vi "RegisterEvents.vi"(8 "Error In":errorcluster, 10 "Root Actor's Enqueuer":refnum<class "Message Enqueuer.lvclass">, 11 "Nested Actor's EnqueuerArray":refnum<class "Message Enqueuer.lvclass">[](array[class])) -> (0 "Error Out":errorcluster)   [LabVIEW 2019, in "TestBench.lvlib" / "TestBench.lvclass"]
uses:
  TestBench.lvclass
  <vilib>/ActorFramework/Message Enqueuer/Message Enqueuer.lvclass
  UserManagement/UserManagement/UserInfo.lvclass
  C:/Program Files (x86)/National Instruments/LabVIEW 2019/vi.lib/NI/Event Source Actor/Event Source/Event/Event.lvclass
  TestBench Messages/SetPrivileges Msg/SetPrivileges Msg.lvclass
  C:/Program Files (x86)/National Instruments/LabVIEW 2019/vi.lib/NI/Event Source Actor/Event Source/Event Source Messages/Event Generated Msg/Event Generated Msg.lvclass
  TestSetup/TestSetup/TestConfiguration.lvclass
  TestBench Messages/Write TestConfiguration Msg/Write TestConfiguration Msg.lvclass
  SoftwareSetup/SoftwareSetup/StationOptions.lvclass
  TestBench Messages/Write StationOptions Msg/Write StationOptions Msg.lvclass
  HardwareSetup_model001/HardwareSetup_modle001/InstrumentCommunication.lvclass
  TestBench Messages/Write InstrumentCommunication Msg/Write InstrumentCommunication Msg.lvclass
  SystemSetup/SystemSetup/SystemConfiguration.lvclass
  TestBench Messages/SystemConfigChanged Msg/SystemConfigChanged Msg.lvclass
  LocalReport/LocalReport/TestReport.lvclass
  TestBench Messages/Write ShortTestReport Msg/Write ShortTestReport Msg.lvclass
  SignalProcessing/SignalProcessing/LunchTest.lvclass
  TestBench Messages/Write Fixture ID Msg/Write Fixture ID Msg.lvclass
  DataBase/DataBase/MySQL initial error.lvclass
  TestBench Messages/Reconnection MySQL Msg/Reconnection MySQL Msg.lvclass
  SignalProcessing/SignalProcessing/Exit.lvclass
  TestBench Messages/Exit Msg/Exit Msg.lvclass
  <vilib>/NI/Event Source Actor/Event Source/Event/Event.lvclass/Event.ctl
  <vilib>/NI/Event Source Actor/Event Source/Event Source Messages/Register Msg/Register Msg.lvclass/Register Msg.ctl
  <vilib>/ActorFramework/Message Enqueuer/Message Enqueuer.lvclass/Message Enqueuer.ctl
  <vilib>/ActorFramework/Message Enqueuer/Enqueue.vi
  <vilib>/NI/Event Source Actor/Event Source/Event Source Messages/Register Msg/Register Msg.lvclass
  C:/Program Files (x86)/National Instruments/LabVIEW 2019/vi.lib/ActorFramework/Message/Message.lvclass
  <vilib>/ActorFramework/Message Priority Queue/Priority Enqueue.vi
  <vilib>/NI/Event Source Actor/Event Source/Event/Event.lvclass
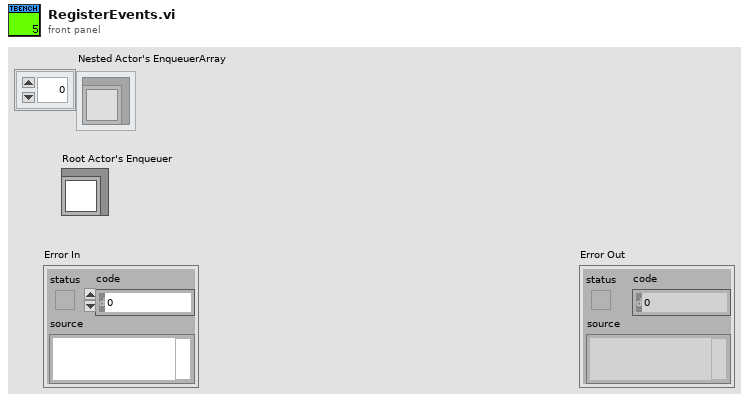
[diagram p1: front panel]
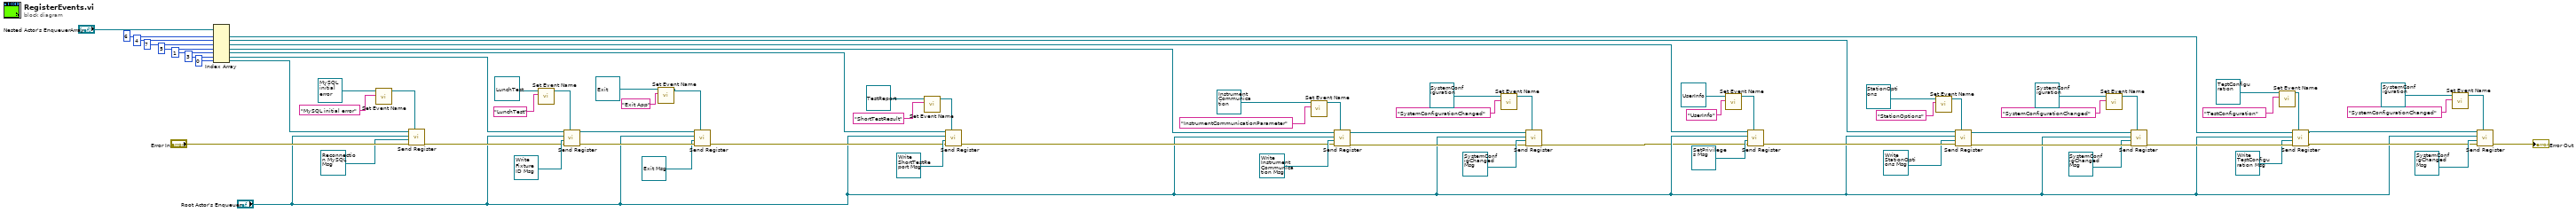
[diagram p0: block diagram]
diagram:
  n1 = Index Array(array="Nested Actor's EnqueuerArray", index #1=6 ("index"), index #2=4 ("index"), index #3=7 ("index"), index #4=5 ("index"), index #5=1 ("index"), index #6=3 ("index"), index #7=0 ("index")) -> (element #1=w67:refnum<class "Message Enqueuer.lvclass">, element #2=w68:refnum<class "Message Enqueuer.lvclass">, element #3=w69:refnum<class "Message Enqueuer.lvclass">, element #4=w4:refnum<class "Message Enqueuer.lvclass">, element #5=w3:refnum<class "Message Enqueuer.lvclass">, element #6=w2:refnum<class "Message Enqueuer.lvclass">, element #7=w1:refnum<class "Message Enqueuer.lvclass">)
  n2 = call <vilib>:"Set Event Name.vi"("Name (Generic)"="MySQL initial error", "Event In"=refnum<class "MySQL initial error.lvclass"> refnum ("DataBase.lvlib:MySQL initial erroe.lvclass")) -> ("Event Out"=w21:refnum<class "MySQL initial error.lvclass">)  [unwired: 9 in]
  n3 = call <vilib>:"Send Register.vi"("Event"=w21, "Error In"="Error In", "Event Handler"=refnum<class "Reconnection MySQL Msg.lvclass"> refnum ("TestBench.lvlib:Reconnection MySQL Msg.lvclass"), "Registrant Address"="Root Actor's Enqueuer", "Event Source Address"=w1) -> ("Error Out"=w19:errorcluster)  [unwired: 5 in, 1 out]
  n4 = call <vilib>:"Set Event Name.vi"("Name (Generic)"="LunchTest", "Event In"=refnum<class "LunchTest.lvclass"> refnum ("SignalProcessing.lvlib:LunchTest.lvclass")) -> ("Event Out"=w25:refnum<class "LunchTest.lvclass">)  [unwired: 9 in]
  n5 = call <vilib>:"Send Register.vi"("Event"=w25, "Error In"=w19, "Event Handler"=refnum<class "Write Fixture ID Msg.lvclass"> refnum ("TestBench.lvlib:Write Fixture ID Msg.lvclass"), "Registrant Address"="Root Actor's Enqueuer", "Event Source Address"=w2) -> ("Error Out"=w16:errorcluster, "Event Source Address Out"=w15:refnum<class "Message Enqueuer.lvclass">)  [unwired: 5 in]
  n6 = call <vilib>:"Set Event Name.vi"("Name (Generic)"="Exit App", "Event In"=refnum<class "Exit.lvclass"> refnum ("SignalProcessing.lvlib:Exit.lvclass")) -> ("Event Out"=w12:refnum<class "Exit.lvclass">)  [unwired: 9 in]
  n7 = call <vilib>:"Send Register.vi"("Event"=w12, "Event Handler"=refnum<class "Exit Msg.lvclass"> refnum ("TestBench.lvlib:Exit Msg.lvclass"), "Registrant Address"="Root Actor's Enqueuer", "Event Source Address"=w15) -> ()  [unwired: 6 in, 2 out]
  n8 = call <vilib>:"Set Event Name.vi"("Name (Generic)"="ShortTestResult", "Event In"=refnum<class "TestReport.lvclass"> refnum ("LocalReport.lvlib:TestReport.lvclass")) -> ("Event Out"=w29:refnum<class "TestReport.lvclass">)  [unwired: 9 in]
  n9 = call <vilib>:"Send Register.vi"("Event"=w29, "Error In"=w16, "Event Handler"=refnum<class "Write ShortTestReport Msg.lvclass"> refnum ("TestBench.lvlib:Write ShortTestReport Msg.lvclass"), "Registrant Address"="Root Actor's Enqueuer", "Event Source Address"=w3) -> ("Error Out"=w17:errorcluster)  [unwired: 5 in, 1 out]
  n10 = call <vilib>:"Set Event Name.vi"("Name (Generic)"="InstrumentCommunicationParameter", "Event In"=refnum<class "InstrumentCommunication.lvclass"> refnum ("HardwareSetup_modle001.lvlib:InstrumentCommunication.lvclass")) -> ("Event Out"=w48:refnum<class "InstrumentCommunication.lvclass">)  [unwired: 9 in]
  n11 = call <vilib>:"Send Register.vi"("Event"=w48, "Error In"=w17, "Event Handler"=refnum<class "Write InstrumentCommunication Msg.lvclass"> refnum ("TestBench.lvlib:Write InstrumentCommunication Msg.lvclass"), "Registrant Address"="Root Actor's Enqueuer", "Event Source Address"=w4) -> ("Error Out"=w33:errorcluster, "Event Source Address Out"=w32:refnum<class "Message Enqueuer.lvclass">)  [unwired: 5 in]
  n12 = call <vilib>:"Set Event Name.vi"("Name (Generic)"="SystemConfigurationChanged", "Event In"=refnum<class "SystemConfiguration.lvclass"> refnum ("SystemSetup.lvlib:SystemConfiguration.lvclass")) -> ("Event Out"=w35:refnum<class "SystemConfiguration.lvclass">)  [unwired: 9 in]
  n13 = call <vilib>:"Send Register.vi"("Event"=w35, "Error In"=w33, "Event Handler"=refnum<class "SystemConfigChanged Msg.lvclass"> refnum ("TestBench.lvlib:SystemConfigChanged Msg.lvclass"), "Registrant Address"="Root Actor's Enqueuer", "Event Source Address"=w32) -> ("Error Out"=w9:errorcluster)  [unwired: 5 in, 1 out]
  n14 = call <vilib>:"Set Event Name.vi"("Name (Generic)"="UserInfo", "Event In"=refnum<class "UserInfo.lvclass"> refnum ("UserManagement.lvlib:UserInfo.lvclass")) -> ("Event Out"=w74:refnum<class "UserInfo.lvclass">)  [unwired: 9 in]
  n15 = call <vilib>:"Send Register.vi"("Event"=w74, "Error In"=w9, "Event Handler"=refnum<class "SetPrivileges Msg.lvclass"> refnum ("TestBench.lvlib:SetPrivileges Msg.lvclass"), "Registrant Address"="Root Actor's Enqueuer", "Event Source Address"=w69) -> ("Error Out"=w66:errorcluster)  [unwired: 5 in, 1 out]
  n16 = call <vilib>:"Set Event Name.vi"("Name (Generic)"="StationOptions", "Event In"=refnum<class "StationOptions.lvclass"> refnum ("SoftwareSetup.lvlib:StationOptions.lvclass")) -> ("Event Out"=w72:refnum<class "StationOptions.lvclass">)  [unwired: 9 in]
  n17 = call <vilib>:"Send Register.vi"("Event"=w72, "Error In"=w66, "Event Handler"=refnum<class "Write StationOptions Msg.lvclass"> refnum ("TestBench.lvlib:Write StationOptions Msg.lvclass"), "Registrant Address"="Root Actor's Enqueuer", "Event Source Address"=w68) -> ("Error Out"=w65:errorcluster, "Event Source Address Out"=w61:refnum<class "Message Enqueuer.lvclass">)  [unwired: 5 in]
  n18 = call <vilib>:"Set Event Name.vi"("Name (Generic)"="SystemConfigurationChanged", "Event In"=refnum<class "SystemConfiguration.lvclass"> refnum ("SystemSetup.lvlib:SystemConfiguration.lvclass")) -> ("Event Out"=w62:refnum<class "SystemConfiguration.lvclass">)  [unwired: 9 in]
  n19 = call <vilib>:"Send Register.vi"("Event"=w62, "Error In"=w65, "Event Handler"=refnum<class "SystemConfigChanged Msg.lvclass"> refnum ("TestBench.lvlib:SystemConfigChanged Msg.lvclass"), "Registrant Address"="Root Actor's Enqueuer", "Event Source Address"=w61) -> ("Error Out"=w64:errorcluster)  [unwired: 5 in, 1 out]
  n20 = call <vilib>:"Set Event Name.vi"("Name (Generic)"="TestConfiguration", "Event In"=refnum<class "TestConfiguration.lvclass"> refnum ("TestSetup.lvlib:TestConfiguration.lvclass")) -> ("Event Out"=w70:refnum<class "TestConfiguration.lvclass">)  [unwired: 9 in]
  n21 = call <vilib>:"Send Register.vi"("Event"=w70, "Error In"=w64, "Event Handler"=refnum<class "Write TestConfiguration Msg.lvclass"> refnum ("TestBench.lvlib:Write TestConfiguration Msg.lvclass"), "Registrant Address"="Root Actor's Enqueuer", "Event Source Address"=w67) -> ("Error Out"=w39:errorcluster, "Event Source Address Out"=w40:refnum<class "Message Enqueuer.lvclass">)  [unwired: 5 in]
  n22 = call <vilib>:"Set Event Name.vi"("Name (Generic)"="SystemConfigurationChanged", "Event In"=refnum<class "SystemConfiguration.lvclass"> refnum ("SystemSetup.lvlib:SystemConfiguration.lvclass")) -> ("Event Out"=w42:refnum<class "SystemConfiguration.lvclass">)  [unwired: 9 in]
  n23 = call <vilib>:"Send Register.vi"("Event"=w42, "Error In"=w39, "Event Handler"=refnum<class "SystemConfigChanged Msg.lvclass"> refnum ("TestBench.lvlib:SystemConfigChanged Msg.lvclass"), "Registrant Address"="Root Actor's Enqueuer", "Event Source Address"=w40) -> ("Error Out"=→"Error Out":errorcluster)  [unwired: 5 in, 1 out]
